vi "MB1010AnalogPID.vi"(5 "output range (100, -100)":cluster{"output high":dbl, "output low":dbl}={"output high"=100.0, "output low"=-100.0} {"output low" format="%.2f"; "output high" format="%.2f"}, 6 "Forward":bool, 7 "PID gains":T4={"proportional gain (Kc)"=1.0, "integral time (Ti, min)"=0.01, "derivative time (Td, min)"=0.0} {"derivative time (Td, min)" format="%.3f"; "integral time (Ti, min)" format="%.3f"; "proportional gain (Kc)" format="%.3f"}, 8 "error in (no error)":errorcluster, 9 "FullSpeed":bool, 10 "setpoint":dbl format="%.2f", 11 "AIDeviceRef":T1={"DevStatus"={"status"=FALSE, "code"=0, "source"=""}, "Controller"=enum."Controller 1", "Analog Channel"=enum."AI 1"}) -> (0 "error out":errorcluster, 1 "CrossedSetpoint":bool, 2 "output":dbl, 3 "AIDeviceRef":T1={"DevStatus"={"status"=FALSE, "code"=0, "source"=""}, "Controller"=enum."Controller 1", "Analog Channel"=enum."AI 1"})   [LabVIEW 2014]
uses:
  <vilib>/Rock Robotics/WPI/AnalogChannel/WPI_AnalogChannelDevRef.ctl
  <vilib>/Rock Robotics/SystemInterfaces/Typedef/FPGA_TypedefAnalogModule.ctl
  <vilib>/Rock Robotics/SystemInterfaces/AI/FPGA_AIChannel.ctl
  <vilib>/addons/control/pid/pid.llb/PID Control Input Filter (DBL).vi
  <vilib>/addons/control/pid/pid.llb/PID (DBL).vi
  <vilib>/addons/control/pid/NI_PID_pid.lvlib
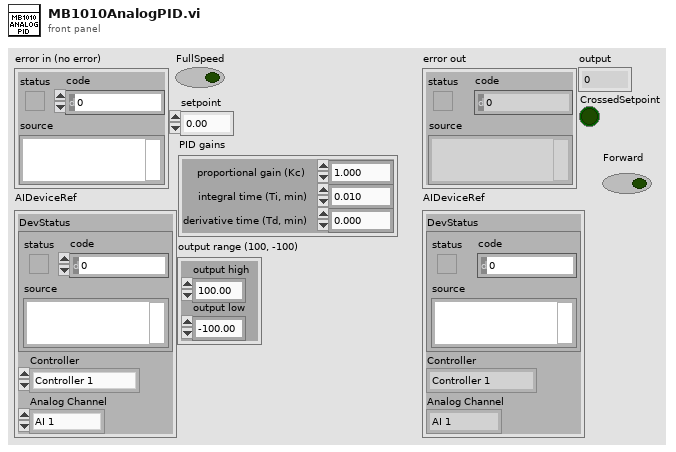
[diagram p1: front panel]
types:
  T1 = typedef "WPI_AnalogChannelDevRef.ctl" = cluster{"DevStatus":errorcluster, "Controller":T2, "Analog Channel":T3}
  T2 = typedef "FPGA_TypedefAnalogModule.ctl" = enum16{"Controller 1"}
  T3 = typedef "FPGA_AIChannel.ctl" = enum8{"AI 0", "AI 1", "AI 2", "AI 3", "AI MXP 0", "AI MXP 1", "AI MXP 2", "AI MXP 3", "Invalid"}
  T4 = cluster{"proportional gain (Kc)":dbl, "integral time (Ti, min)":dbl, "derivative time (Td, min)":dbl}
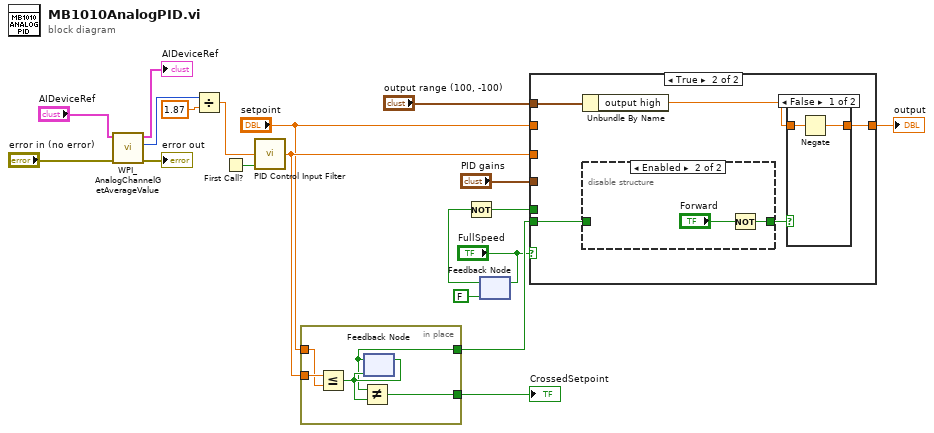
[diagram p0: block diagram]
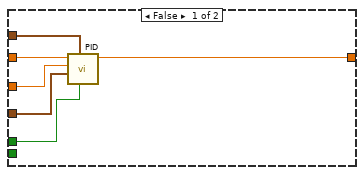
[diagram p2: hidden frame]
diagram:
  n1 = call <vilib>:"WPI_AnalogChannelGetAverageValue.vi"("error in (no error)"="error in (no error)", "AIDeviceRef"="AIDeviceRef") -> ("error out"=→"error out":errorcluster, "Value"=w19:i32, "AIDeviceRef"=→"AIDeviceRef":T1)  [unwired: 7 in]
  n2 = Divide(x=w19, y=1.87 ("scaling factor")) -> (x/y=w18:dbl)
  n3 = First Call?() -> (First Call?: T/F=w1:bool)
  n4 = call-poly <vilib>:"PID Control Input Filter.vi"("reinitialize? (F)"=w1, "input"=w18) -> ("output"=w13:dbl)  [unwired: 3 in]
  n5 = in-place {
    in-place-border: w13 -> [w24]
    in-place-border: [w23] -> w2
    in-place-border: [w21] -> w12
    in-place-border: "setpoint" -> [w20]
    n6 = Less Or Equal?(x=w24, y=w20) -> (x <= y?=w22:bool)
    n7 = feedback #1(w22) -> (w21:bool)
    n8 = Not Equal?(x=w21, y=w22) -> (x != y?=w23:bool)
    n9 = feedback-in #1(w22) -> ()
  }
  "CrossedSetpoint" <- w2
  n10 = feedback #2(FALSE) -> (w14:bool)
  n11 = Not(x=w14) -> (.not. x?=w15:bool)
  n12 = feedback-in #2("FullSpeed") -> ()
  n13 = case shown="True" "FullSpeed" {
    tunnel: w15 -> [w30 _]
    tunnel: [w29 w35] -> w4
    tunnel: w13 -> [w28 _]
    tunnel: w12 -> [_ w31]
    tunnel: "setpoint" -> [w27 _]
    tunnel: "output range (100, -100)" -> [w26 w34]
    tunnel: "PID gains" -> [w25 _]
    frame False {
      n14 = call-poly <vilib>:"PID.vi"("reinitialize? (F)"=w30, "output range"=w26, "PID gains"=w25, "process variable"=w28, "setpoint"=w27) -> ("output"=w29:dbl)  [unwired: 5 in, 1 out]
    }
    frame True {
      n15 = Unbundle By Name(w34) -> ("output high"=w33:dbl)
      n16 = disable-structure shown="Enabled" {
        disable-tunnel: [w36 w37] -> w32
        disable-tunnel: w31 -> [w36 _]
        frame Disabled {
        }
        frame Enabled {
          n17 = Not(x="Forward") -> (.not. x?=w37:bool)
        }
      }
      n18 = case shown="False" w32 {
        tunnel: [w40 w41] -> w35
        tunnel: w33 -> [w39 w41]
        frame False {
          n19 = Negate(x=w39) -> (-x=w40:dbl)
        }
        frame True {
        }
      }
    }
  }
  "output" <- w4
